vi "FieldDisp_Read_Image_File.vi"(11 "file":path) -> (0 "Image Error":errorcluster, 1 "Image Out":T1, 2 "Picture Error":errorcluster, 3 "Picture Data":T2)   [LabVIEW 2019, in "Trajectory_Library.lvlib"]
doc: "Internal function -- should not be called directly by users.\n\nComplete documentation TBD."
uses:
  <vilib>/picture/picture.llb/imagedata.ctl
  <vilib>/vision/Image Controls.llb/IMAQ Image.ctl
  Trajectory_Library.lvlib
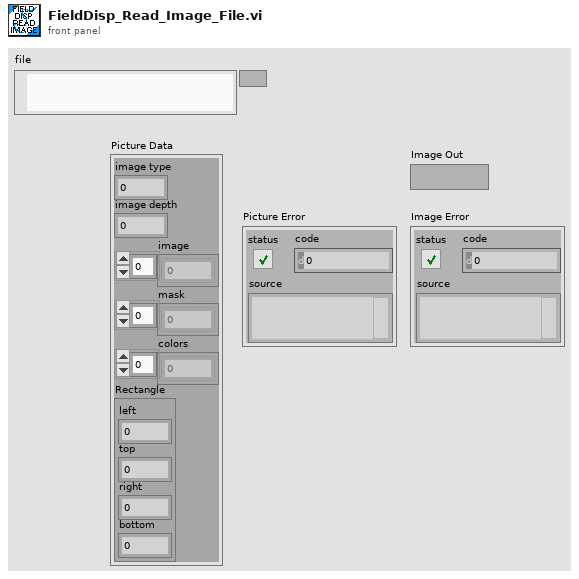
[diagram p1: front panel]
types:
  T1 = typedef "IMAQ Image.ctl" = refnum<image>
  T2 = typedef "imagedata.ctl" = cluster{"image type":i32, "image depth":i32, "image":u8[], "mask":u8[], "colors":u32[], "Rectangle":cluster{"left":i16, "top":i16, "right":i16, "bottom":i16}}
  T3 = typedef "Image Type" = u32
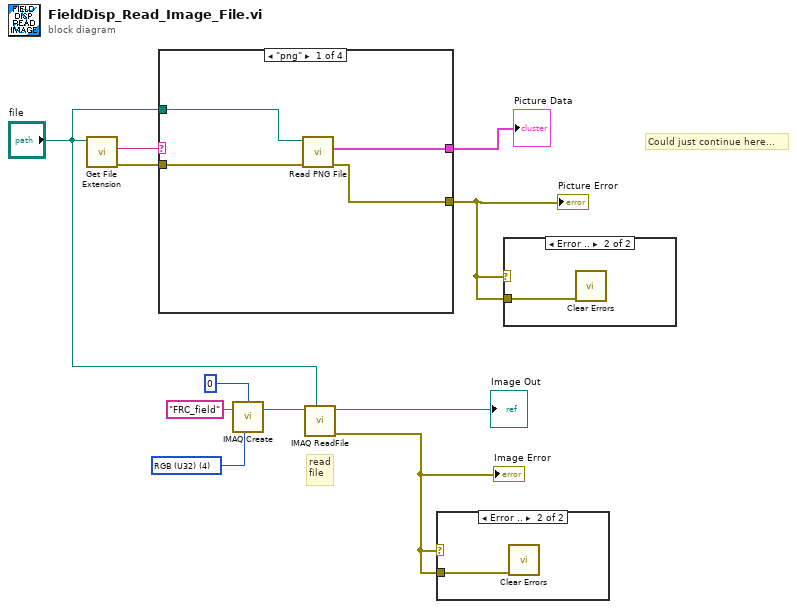
[diagram p0: block diagram]
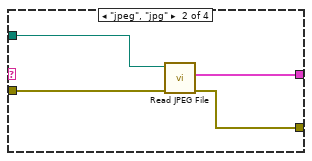
[diagram p4: hidden frame]
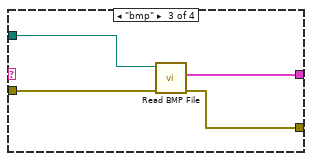
[diagram p5: hidden frame]
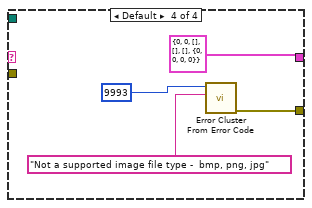
[diagram p6: hidden frame]
diagram:
  w4 = T3 4 items=["Grayscale (U8)", "Grayscale (I16)", "Grayscale (SGL)", "Complex (CSG)", "RGB (U32)", "HSL (U32)", "RGB (U64)", "Grayscale (U16)"] ("Image Type")
  # "read\nfile"
  # "Could just continue here..."
  n1 = call <vilib>:"Get File Extension.vi"("file"="file") -> ("error out"=w8:errorcluster, "lowercase file extension"=w11:string)  [unwired: 6 in, 3 out]
  n2 = case shown="\"png\"" w11 {
    tunnel: "file" -> [w15 w19 w23 _]
    tunnel: [w14 w18 w22 T2 {"image type"=0, "image depth"=0, "image"=[], "mask"=[], "colors"=[], "Rectangle"={"left"=0, "top"=0, "right"=0, "bottom"=0}} ("image data")] -> w10
    tunnel: [w13 w17 w21 w27] -> w2
    tunnel: w8 -> [w12 w16 w20 _]
    frame "png" {
      n3 = call <vilib>:"Read PNG File.vi"("error in (no error)"=w12, "path to PNG file"=w15) -> ("error out"=w13:errorcluster, "image data"=w14:T2)  [unwired: 7 in, 1 out]
    }
    frame "jpeg", "jpg" {
      n4 = call <vilib>:"Read JPEG File.vi"("error in (no error)"=w16, "path to JPEG file"=w19) -> ("error out"=w17:errorcluster, "image data"=w18:T2)  [unwired: 7 in, 1 out]
    }
    frame "bmp" {
      n5 = call <vilib>:"Read BMP File.vi"("error in (no error)"=w20, "path to BMP file"=w23) -> ("error out"=w21:errorcluster, "image data"=w22:T2)  [unwired: 7 in, 1 out]
    }
    frame Default {
      n6 = call <vilib>:"Error Cluster From Error Code.vi"("error message (\"\")"="Not a supported image file type -  bmp, png, jpg" ("error message (\"\")"), "error code (0)"=9993) -> ("error out"=w27:errorcluster)  [unwired: 7 in]
    }
  }
  "Picture Data" <- w10
  "Picture Error" <- w2
  n7 = call "IMAQ Create"("Border Size"=0, "Image Name"="FRC_field", "Image Type"=w4) -> ("New Image"=w6:T1)  [unwired: 2 in, 1 out]
  n8 = call "IMAQ ReadFile"("File Path"="file", "Image"=w6) -> ("error out"=w1:errorcluster, "Image Out"=→"Image Out":T1)  [unwired: 5 in, 3 out]
  "Image Error" <- w1
  n9 = case shown="Error .." w1 {
    tunnel: w1 -> [_ w28]
    frame No Error {
    }
    frame Error {
      n10 = call <vilib>:"Clear Errors.vi"("error in (no error)"=w28) -> ()  [unwired: 5 in, 2 out]
    }
  }
  n11 = case shown="Error .." w2 {
    tunnel: w2 -> [_ w29]
    frame No Error {
    }
    frame Error {
      n12 = call <vilib>:"Clear Errors.vi"("error in (no error)"=w29) -> ()  [unwired: 5 in, 2 out]
    }
  }
